vi "denoise.vi"(7 "Window size":i32, 8 "low cutoff freq: fl (disabled)":dbl=0.12500000000000006 format="%0.4f", 10 "transmissions[r=wl,c=v]":dbl[][](array[numeric]), 11 "voltages":dbl[](array[numeric])) -> (2 "smoothed transmissions[r=wl,c=v]":dbl[][](array[numeric]), 3 "remaining volts":dbl[](array[numeric]))   [LabVIEW 2019]
uses:
  REFS.vi
  <vilib>/Analysis/NI_AALBase.lvlib
  <vilib>/Analysis/3filter.llb/Filter Passband Type.ctl
  <vilib>/Analysis/3filter.llb/Butterworth Filter (DBL).vi
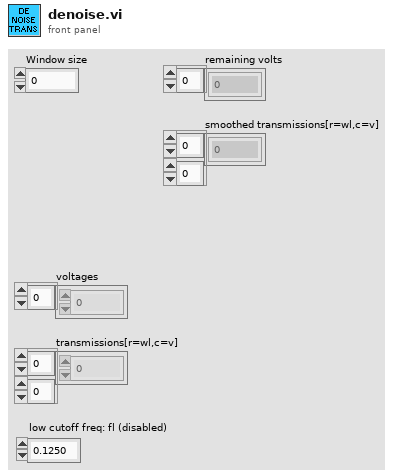
[diagram p1: front panel]
types:
  T1 = typedef "NI_AALBase.lvlib/Filter Passband Type.ctl" = enum32{"Lowpass", "Highpass", "Bandpass", "Bandstop"}
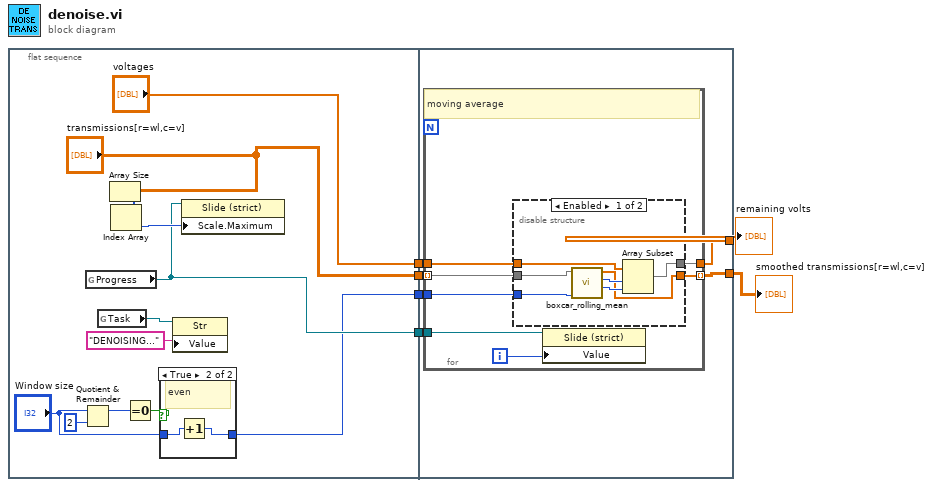
[diagram p0: block diagram]
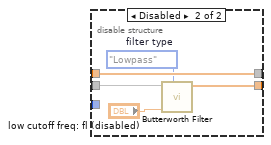
[diagram p3: hidden frame]
diagram:
  n1 = flat-sequence {
    tunnel: [w7] -> w4
    tunnel: ["voltages"] -> w3
    tunnel: [w10] -> w2
    tunnel: ["transmissions[r=wl,c=v]"] -> w1
    tunnel: [w23] -> w6
    tunnel: [w22] -> w5
    tunnel: w4 -> [w27]
    tunnel: w3 -> [w26]
    tunnel: w2 -> [w25]
    tunnel: w1 -> [w24]
    frame #0 {
      n2 = Quotient & Remainder(x="Window size", y=2) -> (x-y*floor(x/y)=w13:i32)  [unwired: 1 out]
      n3 = global read "REFS.vi" "Progress"() -> (w10:refnum<vi>)
      n4 = global read "REFS.vi" "Task"() -> (w16:refnum<vi>)
      n5 = Array Size(array="transmissions[r=wl,c=v]") -> (size(s)=w17:i32[])
      n6 = Index Array(array=w17) -> (element=w18:i32)  [unwired: 1 in]
      n7 = Equal To 0?(x=w13) -> (x = 0?=w14:bool)
      n8 = case shown="True" w14 {
        tunnel: "Window size" -> [w19 w21]
        tunnel: [w19 w20] -> w7
        frame False {
          # "odd"
        }
        frame True {
          # "even"
          n9 = Increment(x=w21) -> (x+1=w20:i32)
        }
      }
      n10 = property class="Str"(reference=w16, "Value"="DENOISING...") -> ()  [unwired: 1 in, 2 out]
      n11 = property on="Property Node" class="Slide (strict)"(reference=w10, "Scale.Maximum"=w18) -> ()  [unwired: 1 in, 2 out]
    }
    frame #1 {
      n12 = for {
        tunnel: w24 -> [w34] mode=indexing
        tunnel: w27 -> [w33]
        tunnel: [w32] -> w23 mode=indexing
        tunnel: [w31] -> w22
        tunnel: w26 -> [w30]
        tunnel: w25 -> [w28]
        i -> [w29]
        # "moving average"
        n13 = disable-structure shown="Enabled" {
          disable-tunnel: w34 -> [w41 w45]
          disable-tunnel: w33 -> [w40 _]
          disable-tunnel: w30 -> [w38 w46]
          disable-tunnel: [w36 w44] -> w32
          disable-tunnel: [w35 w46] -> w31
          frame Enabled {
            n14 = call "boxcar_rolling_mean.vi"("window_width_odd"=w40, "array_in"=w41) -> ("length"=w37:i32, "first_idx"=w39:i32, "array_out"=w36:dbl[])  [unwired: 6 in, 1 out]
            n15 = Array Subset(array=w38, index=w39, length=w37) -> (w35:dbl[])
          }
          frame Disabled {
            w43 = Filter_Passband_Type."Lowpass"  # filter type
            n16 = call-poly <vilib>:"Butterworth Filter.vi"("filter type"=w43, "low cutoff freq: fl"="low cutoff freq: fl (disabled)", "X"=w45) -> ("Filtered X"=w44:dbl[])  [unwired: 5 in, 1 out]
          }
        }
        n17 = property class="Slide (strict)"(reference=w28, "Value"=w29) -> ()  [unwired: 1 in, 2 out]
      }
    }
  }
  "smoothed transmissions[r=wl,c=v]" <- w6
  "remaining volts" <- w5
